vi "ContourManual2010.vi"   [LabVIEW 2013]
uses:
  <vilib>/Heliosphere Research LLC/Advanced Plotting Toolkit/api_plotting/Contour_Manual.vi
  <vilib>/Heliosphere Research LLC/Advanced Plotting Toolkit/Advanced Plotting Toolkit.lvlib
types:
  T1 = typedef "Advanced Plotting Toolkit.lvlib/PlotID.ctl" = i32
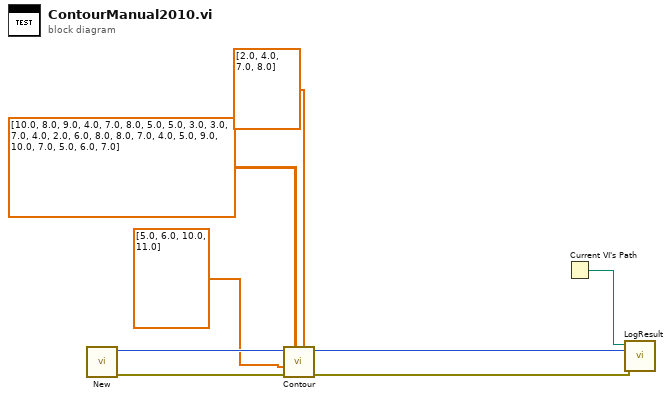
[diagram p0: block diagram]
diagram:
  n1 = call <vilib>:"New.vi"() -> ("error out"=w5:errorcluster, "Plot ID"=w6:T1)  [unwired: 10 in]
  n2 = call-poly <vilib>:"Contour.vi"("Levels"=dbl[] [2.0, 4.0, 7.0, 8.0], "Z Data"=dbl[][] [[10.0, 8.0, 9.0, 4.0, 7.0], [8.0, 5.0, 5.0, 3.0, 3.0], [7.0, 4.0, 2.0, 6.0, 8.0], [8.0, 7.0, 4.0, 5.0, 9.0], [10.0, 7.0, 5.0, 6.0, 7.0]], "error in (no error)"=w5, "Y Coordinates"=dbl[] [5.0, 6.0, 10.0, 11.0] ("X Coordinates"), "Plot ID"=w6) -> ("error out"=w3:errorcluster, "Plot ID Out"=w4:T1)  [unwired: 5 in]
  n3 = Current VI's Path() -> (path=w8:path)
  n4 = call "LogResult.vi"("Test Result"=w3, "Test Artifact"=w4, "VI Path"=w8) -> ()  [unwired: 9 in]
